vi "_Read.vi"(8 "error in (no error)":errorcluster, 11 "Anritsu Optical Power Meter  in":refnum<class "Anritsu Optical Power Meter .lvclass">) -> (0 "error out":errorcluster, 2 "X array":T1, 3 "Anritsu Optical Power Meter  out":refnum<class "Anritsu Optical Power Meter .lvclass">)   [LabVIEW 2012, in "Anritsu Optical Power Meter .lvclass"]
doc: "(Protected, Dynamic, Pure Virtual/Abstract) Perform a measurement and return one or more channels of data. Outsiders should not call this method, but instead the public \"Read Data.vi\"."
uses:
  Anritsu Optical Power Meter .lvclass
  Utility Classes/Readable/X array.ctl
  Utility Classes/Readable/X.ctl
  Utility Classes/Readable/Readable.lvclass
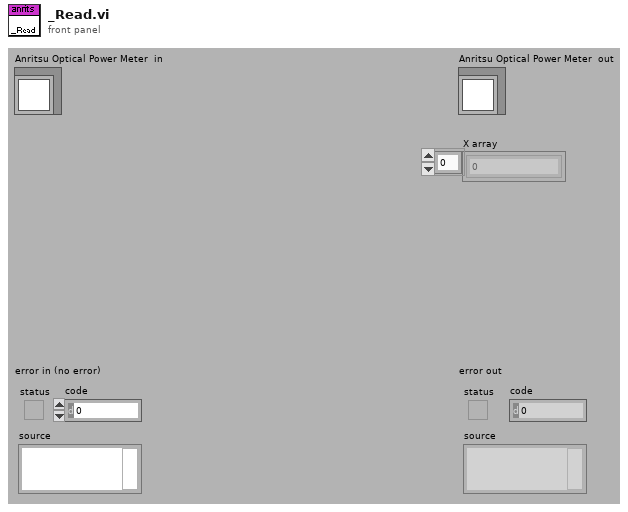
[diagram p1: front panel]
types:
  T1 = typedef "Readable.lvclass/X array.ctl" = T2[]
  T2 = typedef "Readable.lvclass/X.ctl" = dbl
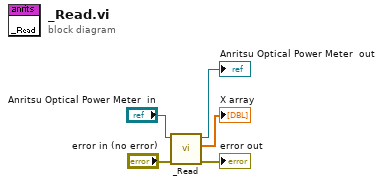
[diagram p0: block diagram]
diagram:
  n1 = call-parent "_Read.vi"("error in (no error)"="error in (no error)", "Readable in"="Anritsu Optical Power Meter  in") -> ("error out"=→"error out":errorcluster, "X array"=→"X array":T1, "Readable out"=→"Anritsu Optical Power Meter  out":refnum<class "Anritsu Optical Power Meter .lvclass">)  [unwired: 7 in]
